vi "take_gentec_photodiode_reading.vi"(5 "numeric array":dbl[](array[numeric])) -> (0 "SD":string, 1 "Mean":string, 2 "Num of readings":string)   [LabVIEW 2020]
panel:
  out "sum":dbl
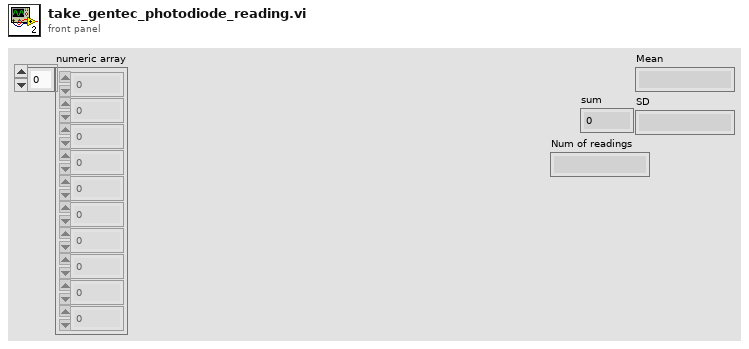
[diagram p1: front panel]
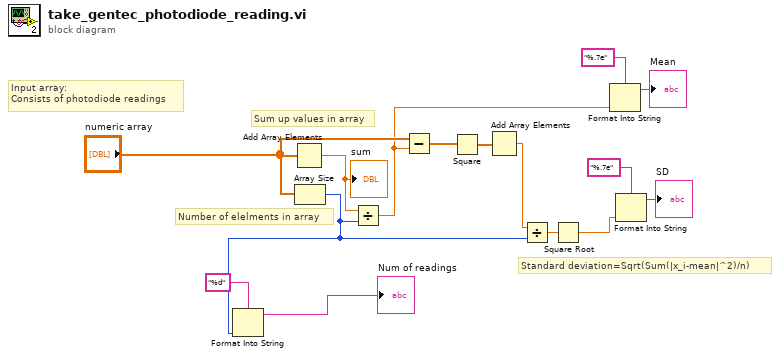
[diagram p0: block diagram]
diagram:
  # "Standard deviation=Sqrt(Sum(|x_i-mean|^2)/n)"
  # "Number of elelments in array"
  # "Sum up values in array"
  # "Input array:\nConsists of photodiode readings"
  n1 = Add Array Elements(numeric array="numeric array") -> (sum=w15:dbl)
  "sum" <- w15
  n2 = Array Size(array="numeric array") -> (size(s)=w3:i32)
  n3 = Format Into String(format string="%d", w3) -> (resulting string=→"Num of readings":string)  [unwired: 2 in, 1 out]
  n4 = Divide(x=w15, y=w3) -> (x/y=w8:dbl)
  n5 = Subtract(x="numeric array", y=w8) -> (x-y=w12:dbl[])
  n6 = Square(x=w12) -> (x^2=w11:dbl[])
  n7 = Add Array Elements(numeric array=w11) -> (sum=w13:dbl)
  n8 = Divide(x=w13, y=w3) -> (x/y=w14:dbl)
  n9 = Square Root(x=w14) -> (sqrt(x)=w6:dbl)
  n10 = Format Into String(format string="%.7e", w8) -> (resulting string=→"Mean":string)  [unwired: 2 in, 1 out]
  n11 = Format Into String(format string="%.7e", w6) -> (resulting string=→"SD":string)  [unwired: 2 in, 1 out]
